vi "UDP Diag.vi"() -> ()   [LabVIEW 2009]
panel:
  out ".not. x?":bool
  out "Timeout":bool
  out "Receive Data":string
  out "error out":errorcluster
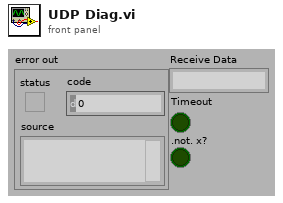
[diagram p1: front panel]
types:
  T1 = typedef "UDP Base.ctl" = cluster{"UDP Session":refnum<k16>, "UDP Socket Params":T2}
  T2 = typedef "UDP Socket Params.ctl" = cluster{"Local Port":u16, "Read Timeout":i32, "Write Timeout":i32}
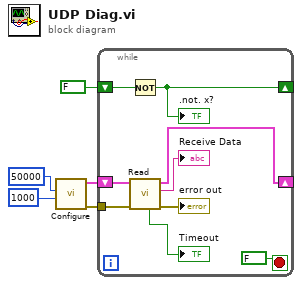
[diagram p0: block diagram]
diagram:
  n1 = call "Configure.vi"("Read Timeout"=1000, "Local Port"=u16 50000) -> ("error out"=w4:errorcluster, "UDP Base out"=w5:T1)  [unwired: 8 in]
  n2 = while {
    tunnel: w4 -> [w13]
    shift-right: [w12] -> _
    shift-left: w5 -> [w14]
    shift-right: [w6] -> _
    shift-left: FALSE ("Timeout") -> [w7]
    stop <- FALSE stop-if-true
    n3 = Not(x=w7) -> (.not. x?=w6:bool)
    ".not. x?" <- w6
    n4 = call "Read.vi"("error in (no error)"=w13, "UDP Base in"=w14) -> ("error out"=→"error out":errorcluster, "Receive Data"=→"Receive Data":string, "UDP Base out"=w12:T1, "Timeout"=→"Timeout":bool)  [unwired: 4 in, 2 out]
  }
